vi "SE_HV200.ProcConstructor.vi"(0 "i ref in":refnum<vi>, 5 "error in (no error)":errorcluster) -> (14 "i ref out":refnum<vi>, 19 "error out":errorcluster)   [LabVIEW 2014, in "SE_HV200.lvlib"]
doc: "This method allows to do initialization (to serve as a constructor for attributes). It is necessary, since the BaseProcess.i attribute is not initialized when the ClassName.constructor is executed."
uses:
  SE_HV200.lvlib
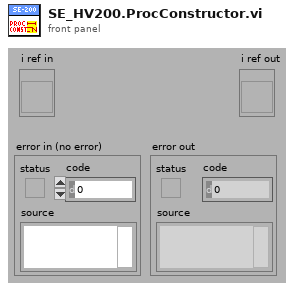
[diagram p1: front panel]
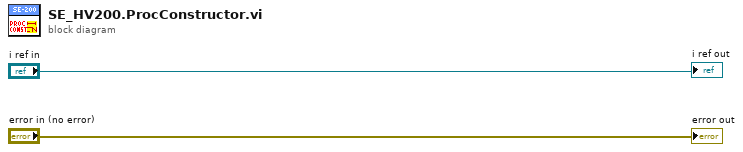
[diagram p0: block diagram]
diagram:
  "error out" <- "error in (no error)"
  "i ref out" <- "i ref in"
